vi "写入光源亮度.vi"(8 "错误输入（无错误）":errorcluster, 10 "光源亮度":T1, 11 "下拉列表":u16) -> (0 "错误输出":errorcluster)   [LabVIEW 2017]
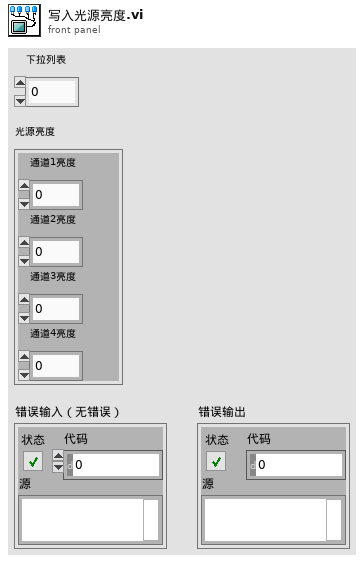
[diagram p1: front panel]
types:
  T1 = cluster{"通道1亮度":u32, "通道2亮度":u32, "通道3亮度":u32, "通道4亮度":u32}
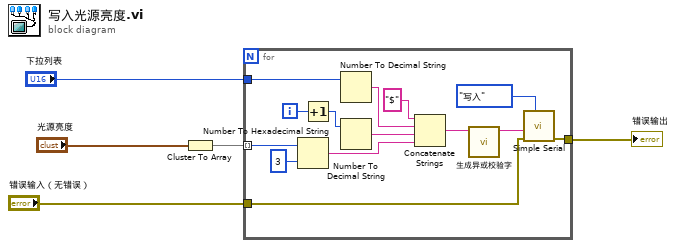
[diagram p0: block diagram]
diagram:
  n1 = Cluster To Array(cluster="光源亮度") -> (array=w2:u32[])
  n2 = for {
    tunnel: w2 -> [w18] mode=indexing
    tunnel: "下拉列表" -> [w17]
    tunnel: [w7] -> w5
    tunnel: "错误输入（无错误）" -> [w6]
    i -> [w14]
    n3 = Number To Hexadecimal String(1:i16 3 ("宽度(-)"), 2:w18) -> (0:w10:string)
    n4 = Increment(x=w14) -> (x+1=w13:i32)
    n5 = Number To Decimal String(number=w17) -> (decimal integer string=w15:string)  [unwired: 1 in]
    n6 = Number To Decimal String(number=w13) -> (decimal integer string=w12:string)  [unwired: 1 in]
    n7 = Concatenate Strings("$", w15, w12, w10) -> (w9:string)
    n8 = call "生成异或校验字.vi"("字符串"=w9) -> ("连接的字符串"=w8:string)  [unwired: 9 in, 1 out]
    n9 = call "Simple Serial.vi"("选项"=enum16{"打开", "写入", "读取", "关闭"}."写入", "error in"=w6, "写入缓冲区"=w8) -> ("error out"=w7:errorcluster)  [unwired: 6 in, 2 out]
  }
  "错误输出" <- w5
